vi "Special_Processing.vi"(6 "cluster in":T1, 8 "error in (no error)":errorcluster, 9 "Terminal Map In":map{string, T3}(c390), 10 "Wires":T2[](array[typedef]), 11 "Node in":refnum<class "Node.lvclass">) -> (0 "error out":errorcluster, 1 "Terminal Map Out":map{string, T3}(c390), 2 "Wires out":T2[](array[typedef]), 3 "Node out":refnum<class "Node.lvclass">)   [LabVIEW 2025, in "Node.lvclass"]
uses:
  Node.lvclass
  wire.ctl
  Terminal.ctl
  bd.ctl
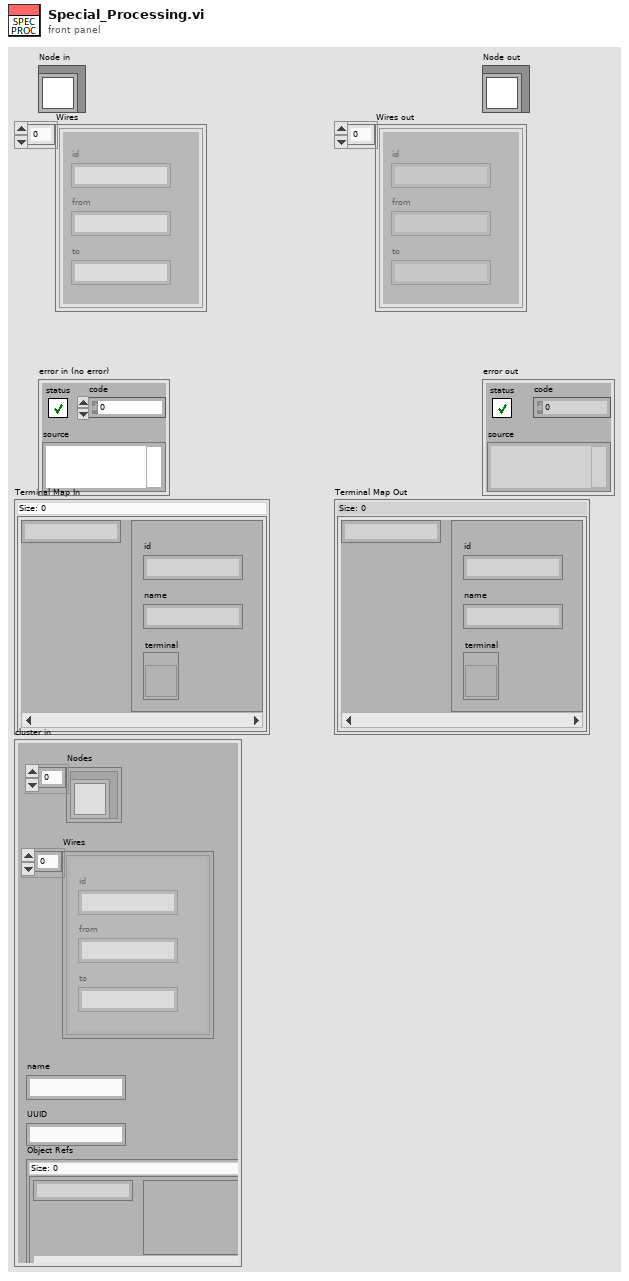
[diagram p1: front panel]
types:
  T1 = typedef "bd.ctl" = cluster{"Nodes":refnum<class "Node.lvclass">[], "Wires":T2[], "name":string, "UUID":string, "Object Refs":map{string, variant}}
  T2 = typedef "wire.ctl" = cluster{"id":string, "from":string, "to":string}
  T3 = typedef "Terminal.ctl" = cluster{"id":string, "name":string, "terminal":refnum<vi>}
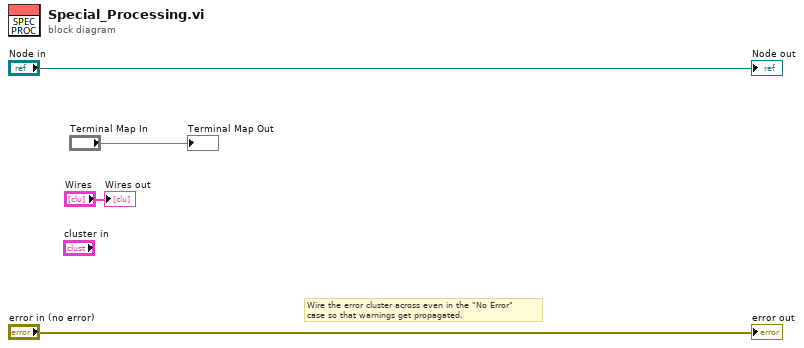
[diagram p0: block diagram]
diagram:
  # "Wire the error cluster across even in the \"No Error\"\ncase so that warnings get propagated."
  "error out" <- "error in (no error)"
  "Node out" <- "Node in"
  "Wires out" <- "Wires"
  "Terminal Map Out" <- "Terminal Map In"
